vi "ConfigPhases.vi"(8 "error in (no error)":errorcluster, 11 "PacificPowerSource in":refnum<class "PacificPowerSource.lvclass">) -> (0 "error out":errorcluster, 3 "PacificPowerSource out":refnum<class "PacificPowerSource.lvclass">)   [LabVIEW 2018, in "AcPwrPlugins.lvlib" / "PacificPowerSource.lvclass"]
doc: "This VI sets the selected logical instrument to apply changes at the set phase angle when operating with synchronization enabled using Configure Synchronization.vi."
uses:
  PacificPowerSource.lvclass
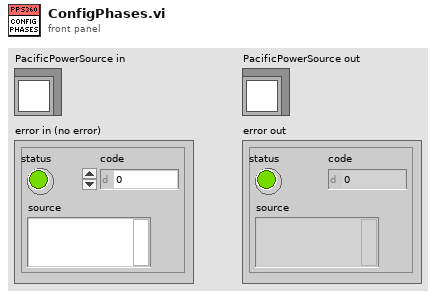
[diagram p1: front panel]
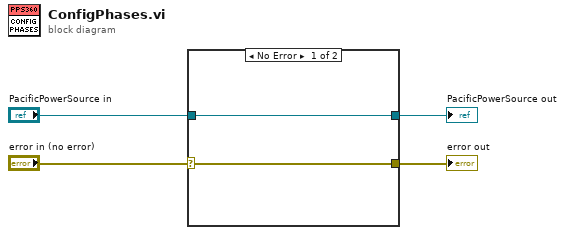
[diagram p0: block diagram]
diagram:
  n1 = case shown="No Error" "error in (no error)" {
    selector: "error in (no error)" -> [w6 w8]
    tunnel: [w6 w8] -> w4
    tunnel: [w5 w7] -> w3
    tunnel: "PacificPowerSource in" -> [w5 w7]
    frame No Error {
    }
    frame Error {
    }
  }
  "error out" <- w4
  "PacificPowerSource out" <- w3
